vi "EditorPDF setParam.vi"(8 "error in (no error)":errorcluster, 10 "Parameter":T3={"Details"={"Title"="", "Subject"="", "Keywords"="", "Author"=""}, "Header/Footer"={"Header"="", "Footer"=""}, "Standard Page"={"Page Size"=10, "Portrait (T:Yes)"=TRUE}} {"Standard Page"."Page Size" items=["LETTER", "NOTE", "LEGAL", "TABLOID", "EXECUTIVE", "POSTCARD", "A0", "A1", "A2", "A3", "A4", "A5", "A6", "A7", "A8", "A9", "A10", "B0", "B1", "B2", "B3", "B4", "B5", "B6", "B7", "B8", "B9", "B10", "ARCH_E", "ARCH_D", "ARCH_C", "ARCH_B", "ARCH_A", "FLSA", "FLSE", "HALFLETTER", "_11X17", "ID_1", "ID_2", "ID_3", "LEDGER", "CROWN_QUARTO", "LARGE_CROWN_QUARTO", "DEMY_QUARTO", "ROYAL_QUARTO", "CROWN_OCTAVO", "LARGE_CROWN_OCTAVO", "DEMY_OCTAVO", "ROYAL_OCTAVO", "SMALL_PAPERBACK", "PENGUIN_SMALL_PAPERBACK", "PENGUIN_LARGE_PAPERBACK"]}, 11 "CreatePDF in":refnum<class "CreatePDF.lvclass">) -> (0 "error out":errorcluster, 3 "CreatePDF out":refnum<class "CreatePDF.lvclass">)   [LabVIEW 2018, in "CreatePDF.lvclass"]
uses:
  CreatePDF.lvclass
  <vilib>/Simplicity AI/SAI_PDF_API/Classes/Context/Controls/SAI_PDF_StdPageLayout.ctl
  <vilib>/Simplicity AI/SAI_PDF_API/Classes/Context/Controls/SAI_PDF_StdPageSize.ctl
  CreatePDF.lvclass/CreatePDF.ctl
  <vilib>/Simplicity AI/SAI_PDF_API/Classes/Context/Context.lvclass
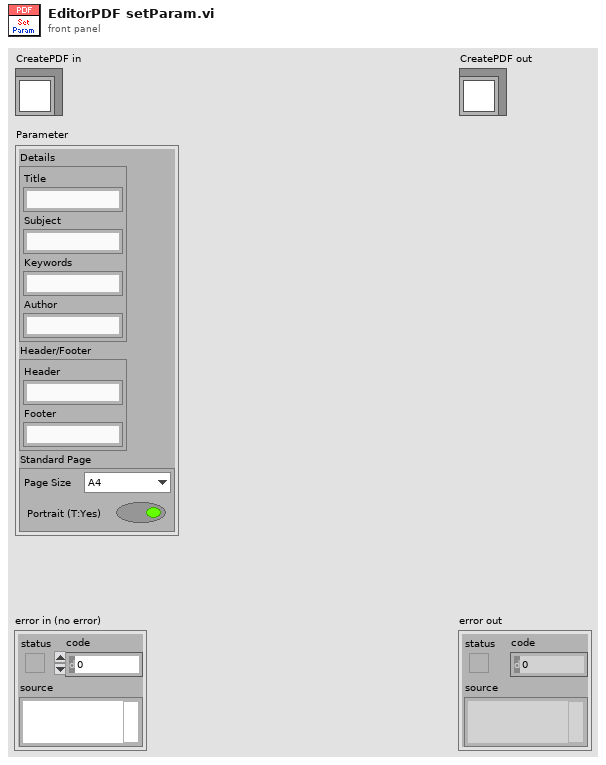
[diagram p1: front panel]
types:
  T1 = typedef "SAI_PDF_Toolkit.lvlib/Context.lvclass/SAI_PDF_StdPageLayout.ctl" = cluster{"Page Size":T2, "Portrait (T:Yes)":bool}
  T2 = typedef "SAI_PDF_Toolkit.lvlib/Context.lvclass/SAI_PDF_StdPageSize.ctl" = i32
  T3 = cluster{"Details":cluster{"Title":string, "Subject":string, "Keywords":string, "Author":string}, "Header/Footer":cluster{"Header":string, "Footer":string}, "Standard Page":T1}
  T4 = cluster{"Title":string, "Subject":string, "Keywords":string, "Author":string}
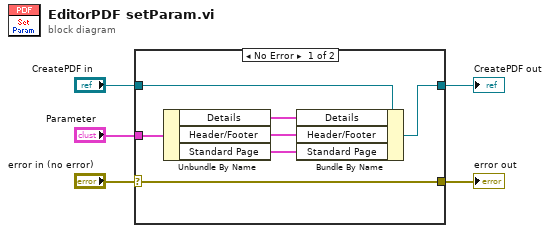
[diagram p0: block diagram]
diagram:
  n1 = case shown="No Error" "error in (no error)" {
    selector: "error in (no error)" -> [w12 w14]
    tunnel: [w12 w14] -> w4
    tunnel: [w6 w13] -> w2
    tunnel: "CreatePDF in" -> [w11 w13]
    tunnel: "Parameter" -> [w10 _]
    frame No Error {
      n2 = Unbundle By Name(w10) -> ("Details"=w9:T4, "Header/Footer"=w8:cluster{"Header":string, "Footer":string}, "Standard Page"=w7:T1)
      n3 = Bundle By Name(cluster=w11, "Details"=w9, "Header/Footer"=w8, "Standard Page"=w7) -> (w6:refnum<class "CreatePDF.lvclass">)
    }
    frame Error {
    }
  }
  "error out" <- w4
  "CreatePDF out" <- w2
